vi "ConfigureSnapshot.vi"(0 "object in":refnum<class "Hamamatsu.lvclass">, 5 "error in (no error)":errorcluster) -> (14 "object out":refnum<class "Hamamatsu.lvclass">, 19 "error out":errorcluster)   [LabVIEW 2021, in "Hamamatsu.lvclass"]
uses:
  Hamamatsu.lvclass
  Hamamatsu.lvclass/Hamamatsu.ctl
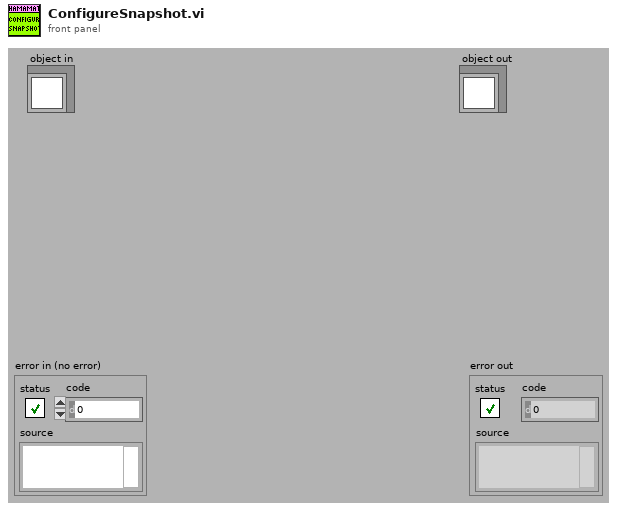
[diagram p1: front panel]
types:
  T1 = typedef "IMAQ Image.ctl" = refnum<image>
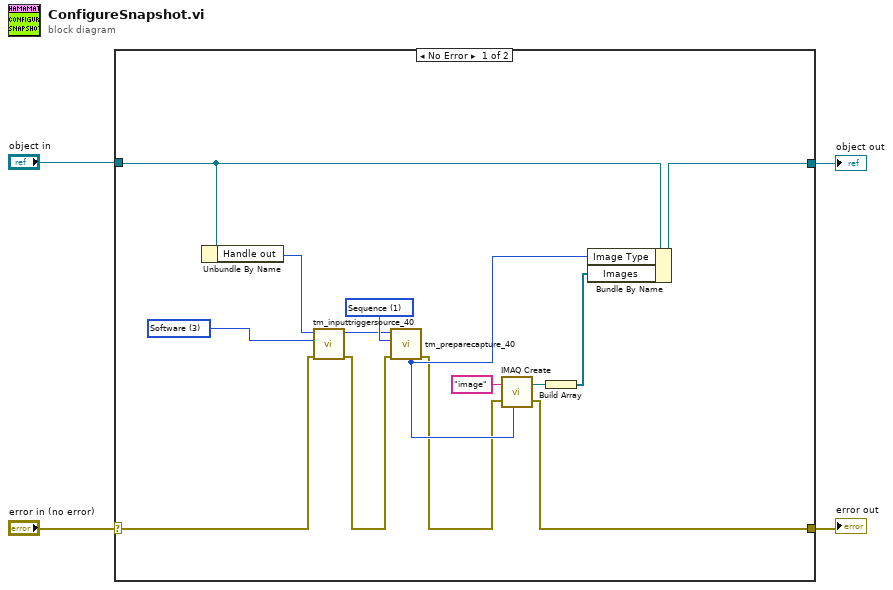
[diagram p0: block diagram]
diagram:
  n1 = case shown="No Error" "error in (no error)" {
    selector: "error in (no error)" -> [w9 w20]
    tunnel: [w13 w20] -> w3
    tunnel: [w17 w19] -> w1
    tunnel: "object in" -> [w18 w19]
    frame No Error {
      w7 = 3 items=["Internal"=1, "External"=2, "Software"=3, "Master Pulse"=4] ("Source")
      w16 = 1 items=["Snap", "Sequence"] ("Capture mode")
      n2 = Unbundle By Name(w18) -> ("Handle out"=w11:u32)
      n3 = call <userlib>:"tm_inputtriggersource_40.vi"("error in (no error)"=w9, "Source"=w7, "Handle in"=w11) -> ("error out"=w8:errorcluster, "Handle out"=w10:u32)  [unwired: 7 in]
      n4 = call <userlib>:"tm_preparecapture_40.vi"("error in (no error)"=w8, "Capture mode"=w16, "Handle in"=w10) -> ("error out"=w12:errorcluster, "Image type"=w14:u32)  [unwired: 5 in, 2 out]
      n5 = call "IMAQ Create"("Image Name"="image", "Image Type"=w14, "error in (no error)"=w12) -> ("New Image"=w6:T1, "error out"=w13:errorcluster)  [unwired: 2 in]
      n6 = Build Array(w6) -> (w5:T1[])
      n7 = Bundle By Name(cluster=w18, "Image Type"=w14, "Images"=w5) -> (w17:refnum<class "Hamamatsu.lvclass">)
    }
    frame Error {
    }
  }
  "error out" <- w3
  "object out" <- w1
